vi "Read ADXL345.vi"(8 "Error In":errorcluster, 10 "Port":i8, 11 "FPGA VI Reference In":T1) -> (0 "error out":errorcluster, 3 "FPGA VI Reference Out":T1, 5 "Y":dbl, 6 "Z":dbl, 7 "X":dbl)   [LabVIEW 2014]
uses:
  Controls/SPI Configuration Cluster.ctl
  Controls/FPGA Reference.ctl
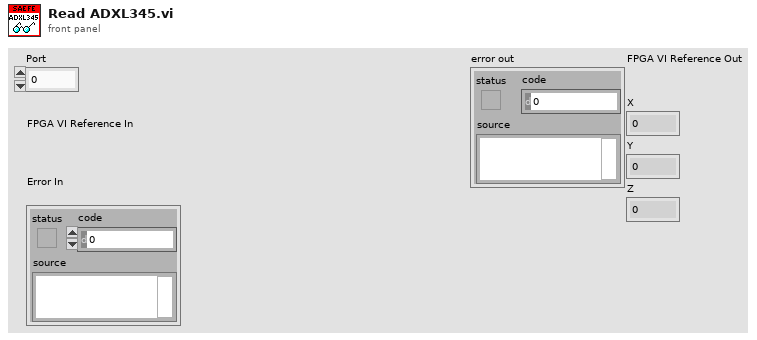
[diagram p1: front panel]
types:
  T1 = typedef "FPGA Reference.ctl" = refnum<k20>
  T2 = typedef "SPI Configuration Cluster.ctl" = cluster{"CS":u8, "Clock Rate (Hz)":dbl, "Clock Mode":u8, "CS Active State":bool}
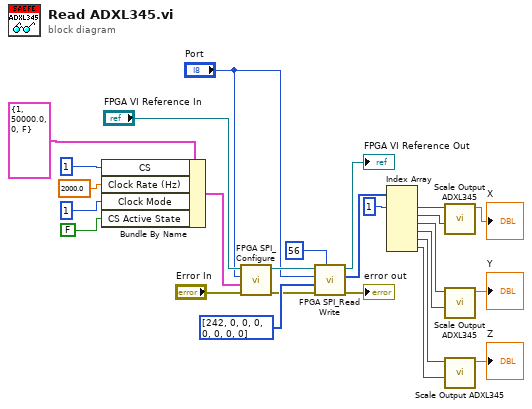
[diagram p0: block diagram]
diagram:
  n1 = Bundle By Name(cluster=T2 {"CS"=1, "Clock Rate (Hz)"=50000.0, "Clock Mode"=0, "CS Active State"=FALSE} ("Configuration Cluster"), "CS"=u8 1, "Clock Rate (Hz)"=2000.0, "Clock Mode"=u8 1, "CS Active State"=FALSE) -> (w6:T2)
  n2 = call "FPGA SPI_Configure.vi"("error in"="Error In", "Configuration Cluster"=w6, "Port"="Port", "FPGA VI Reference"="FPGA VI Reference In") -> ("error out"=w11:errorcluster, "FPGA VI Reference Out"=w10:T1)  [unwired: 5 in, 1 out]
  n3 = call "FPGA SPI_Read Write.vi"("Total Bits"=u16 56, "error in"=w11, "Write Data"=u8[] [242, 0, 0, 0, 0, 0, 0, 0], "Port"="Port", "FPGA VI Reference"=w10) -> ("error out"=→"error out":errorcluster, "Read Data"=w22:u8[], "FPGA VI Reference Out"=→"FPGA VI Reference Out":T1)  [unwired: 4 in]
  n4 = Index Array(array=w22, index #1=1 ("index")) -> (element #1=w20:u8, element #2=w19:u8, element #3=w18:u8, element #4=w17:u8, element #5=w16:u8, element #6=w15:u8)  [unwired: 5 in]
  n5 = call "Scale Output ADXL345.vi"("Byte1"=w19, "Byte0"=w20) -> ("G's"=→"X":fxp<+/-,32,10>)  [unwired: 9 in]
  n6 = call "Scale Output ADXL345.vi"("Byte1"=w17, "Byte0"=w18) -> ("G's"=→"Y":fxp<+/-,32,10>)  [unwired: 9 in]
  n7 = call "Scale Output ADXL345.vi"("Byte1"=w15, "Byte0"=w16) -> ("G's"=→"Z":fxp<+/-,32,10>)  [unwired: 9 in]
